vi "PI_E710_Communicate.vi"(8 "error out 2":errorcluster, 10 "System no.":i32, 11 "String to send":string) -> (0 "error out":errorcluster, 3 "String read":string)   [LabVIEW 2009]
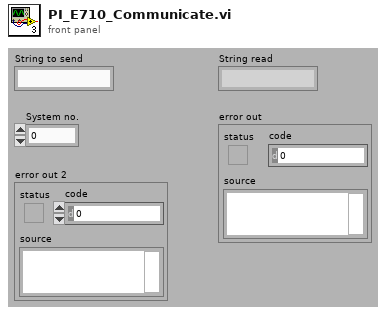
[diagram p1: front panel]
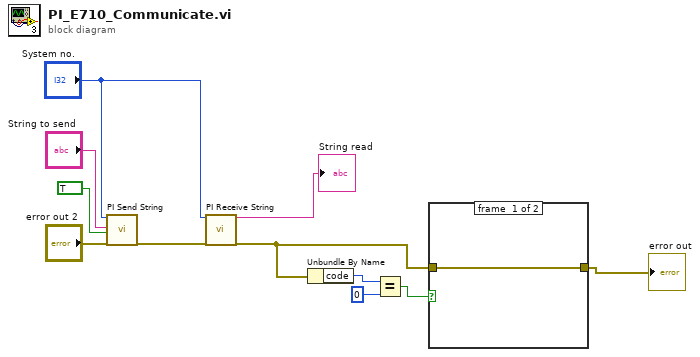
[diagram p0: block diagram]
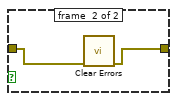
[diagram p2: hidden frame]
diagram:
  n1 = call <userlib>:"PI Send String.vi"("System no."="System no.", "String to send"="String to send", "Attach Linefeed?"=TRUE, "error in"="error out 2") -> ("error out"=w7:errorcluster)  [unwired: 15 out]
  n2 = call <userlib>:"PI Receive String.vi"("System no."="System no.", "error in"=w7) -> ("String read"=→"String read":string, "error out"=w2:errorcluster)  [unwired: 16 out]
  n3 = Unbundle By Name(w2) -> ("code"=w5:i32)
  n4 = Equal?(x=w5, y=0) -> (x = y?=w3:bool)
  n5 = case shown="True" w3 {
    tunnel: w2 -> [w12 w14]
    tunnel: [w12 w13] -> w1
    frame #0 {
    }
    frame #1 {
      n6 = call <vilib>:"Clear Errors.vi"("error in (no error)"=w14) -> ("error out"=w13:errorcluster)  [unwired: 6 in]
    }
  }
  "error out" <- w1
